vi "Test MoveBlock.vi"() -> ()   [LabVIEW 2020, in "sqlite3.lvlib"]
uses:
  sqlite3.lvlib
  5399b6e5-fef8-4e42-8d32-508232ebb59d.vi
  38221cee-6cec-4ecb-b4f6-42b7e8021388.vi
  b4db1361-148b-4e1a-a077-9c5101be366f.vi
panel:
  in  "Array 2":i64[](array[numeric])
  out "Value 4":i64[](array[numeric])
  out "Value 3":dbl[](array[numeric])
  in  "Array":dbl[](array[numeric])
  in  "Numeric Control":u8[](array[numeric])
  out "Value":u8[](array[numeric])
  # "mock up of the malleable VI to test\ndifferent datatypes in edit time.\n\nTesting with a proper CLFN pointer is needed too!"
  # "moveblock is almost exclusively used to dereference binary arrays\nstrings are U8 arrays, etc"
  # "change these datatypes:"
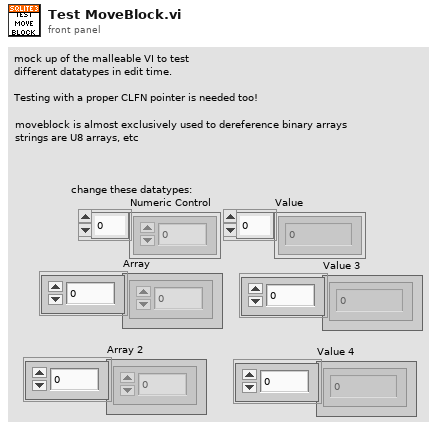
[diagram p1: front panel]
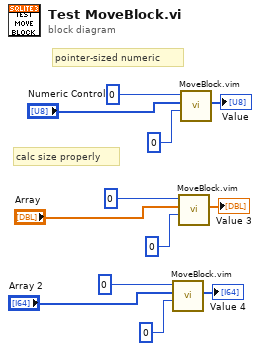
[diagram p0: block diagram]
diagram:
  # "pointer-sized numeric"
  # "calc size properly"
  n1 = call "MoveBlock.vim"("size"=0, "destination (type)"="Array 2", "Address (pointer)"=i64 0) -> ("Value"=→"Value 4":i64[])  [unwired: 7 in, 1 out]
  n2 = call "MoveBlock.vim"("size"=0, "destination (type)"="Array", "Address (pointer)"=i64 0) -> ("Value"=→"Value 3":dbl[])  [unwired: 7 in, 1 out]
  n3 = call "MoveBlock.vim"("size"=0, "destination (type)"="Numeric Control", "Address (pointer)"=i64 0) -> ("Value"=→"Value":u8[])  [unwired: 7 in, 1 out]
